vi "getdrive joystick.vi"(11 "Robot field orientation (deg)":dbl) -> (2 "drive joystick buttons":bool[](array[boolean]), 3 "drive joystick values":dbl[](array[numeric]))   [LabVIEW 2018]
uses:
  <vilib>/Rock Robotics/Network Tables/NT Write Numeric Array.vi
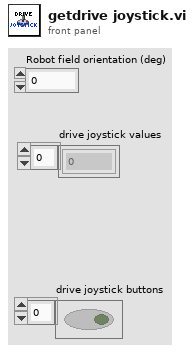
[diagram p1: front panel]
types:
  T1 = typedef "DriveJoystickButtonMapping.ctl" = cluster{"relative encoders?":bool, "zero relative encoder":bool, "reset field orientation":bool, "use field orientation":bool, "braking":bool, "lock rotation":bool}
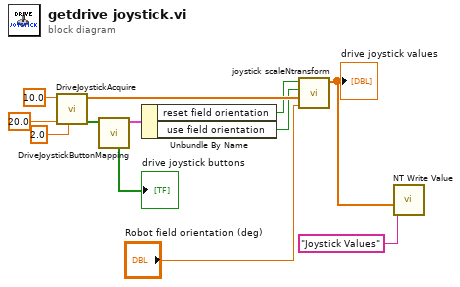
[diagram p0: block diagram]
diagram:
  n1 = call "DriveJoystickAcquire.vi"("Precision Scaler"=2.0, "Rotation Joystick Deadband %"=20.0, "XY Joystick Deadband %"=10.0) -> ("Drive Joystick Buttons"=w8:bool[], "Drive Joystick Values"=w9:dbl[])  [unwired: 7 in]
  n2 = call "DriveJoystickButtonMapping.vi"("drive joystick buttons"=w8) -> ("output cluster"=w6:T1, "drive joystick buttons indicator"=→"drive joystick buttons":bool[])  [unwired: 9 in]
  n3 = Unbundle By Name(w6) -> ("reset field orientation"=w5:bool, "use field orientation"=w4:bool)
  n4 = call "joystick scaleNtransform.vi"("robot field orientation (deg)"="Robot field orientation (deg)", "joystick values"=w9, "use filed orientation"=w4, "reset field orientation"=w5) -> ("Transformed joystick values"=w3:dbl[])  [unwired: 7 in]
  "drive joystick values" <- w3
  n5 = call-poly <vilib>:"NT Write Value.vi"("Numeric Array"=w3, "Name"="Joystick Values") -> ()  [unwired: 9 in, 1 out]
